vi "subFindItemInProject.vi"(9 "Destination path":path, 10 "Source path":path, 11 "TargetItem in":refnum<vi>) -> (0 "error out":errorcluster, 2 "GetProjectItemRefForFile":refnum<vi>, 3 "TargetItem out":refnum<vi>)   [LabVIEW 2019, in "SolutionBuilder.lvlib" / "BuildManager.lvclass"]
uses:
  BuildManager.lvclass
  SolutionBuilder.lvlib
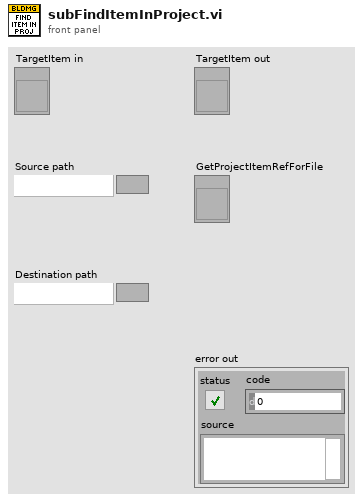
[diagram p1: front panel]
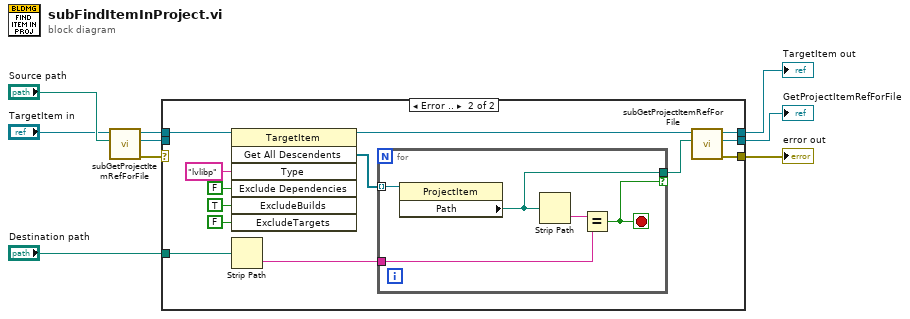
[diagram p0: block diagram]
diagram:
  n1 = call "subGetProjectItemRefForFile.vi"("Source path"="Source path", "TargetItem in"="TargetItem in") -> ("error out"=w7:errorcluster, "GetProjectItemRefForFile"=w3:refnum<vi>, "TargetItem out"=w5:refnum<vi>)  [unwired: 7 in]
  n2 = case shown="Error .." w7 {
    selector: w7 -> [w10 _]
    tunnel: [w12 w15] -> w6
    tunnel: w5 -> [w12 w25]
    tunnel: [w11 w14] -> w4
    tunnel: w3 -> [w11 _]
    tunnel: [w10 w13] -> w2
    tunnel: "Destination path" -> [_ w20]
    frame No Error {
    }
    frame Error {
      n3 = invoke class="TargetItem" method="Get All Descendents"(reference=w25, "Type"="lvlibp", "Exclude Dependencies"=FALSE ("ExcludeDependencies"), "ExcludeBuilds"=TRUE, "ExcludeTargets"=FALSE) -> (reference out=w17:refnum<vi>, "All Descendents"=w19:refnum<vi>[])  [unwired: 2 in, 5 out]
      n4 = Strip Path(path=w20) -> (name=w18:string)  [unwired: 1 out]
      n5 = for {
        tunnel: w19 -> [w30] mode=indexing
        tunnel: w18 -> [w28]
        tunnel: [w26] -> w16 if=w27
        stop <- w27 stop-if-true
        n6 = property class="ProjectItem"(reference=w30) -> ("Path"=w26:path)  [unwired: 1 in, 2 out]
        n7 = Strip Path(path=w26) -> (name=w29:string)  [unwired: 1 out]
        n8 = Equal?(x=w29, y=w28) -> (x = y?=w27:bool)
      }
      n9 = call "subGetProjectItemRefForFile.vi"("Source path"=w16, "TargetItem in"=w17) -> ("error out"=w13:errorcluster, "GetProjectItemRefForFile"=w14:refnum<vi>, "TargetItem out"=w15:refnum<vi>)  [unwired: 7 in]
    }
  }
  "TargetItem out" <- w6
  "error out" <- w2
  "GetProjectItemRefForFile" <- w4
